vi "Joystick Read 1.vi"   [LabVIEW 2011]
uses:
  Robot Global Data.vi
types:
  T1 = typedef "WPI_JoystickDevRef.ctl" = cluster{"Device":T2}
  T2 = typedef "WPI_JoystickDeviceEnum.ctl" = enum16{"USB 1", "USB 2", "USB 3", "USB 4", "Kinect 1", "Kinect 2"}
  T3 = typedef "WPI_JoystickButtonState.ctl" = cluster{"Button 1":bool, "Button 2":bool, "Button 3":bool, "Button 4":bool, "Button 5":bool, "Button 6":bool, "Button 7":bool, "Button 8":bool, "Button 9":bool, "Button 10":bool, "Button 11":bool, "Button 12":bool}
  T4 = cluster{"axis 1 (x)":dbl, "axis 2 (y)":dbl, "axis 3 (throttle)":dbl, "axis 4":dbl, "axis 5":dbl, "axis 6":dbl}
  T5 = cluster{"Axis 1":dbl, "Axis 2":dbl, "Axis 3":dbl, "Axis 4":dbl, "Axis 5":dbl, "Axis 6":dbl, "Button 1":bool, "Button 2":bool, "Button 3":bool, "Button 4":bool, "Button 5":bool, "Button 6":bool, "Button 7":bool, "Button 8":bool, "Button 9":bool, "Button 10":bool, "Button 11":bool, "Button 12":bool}
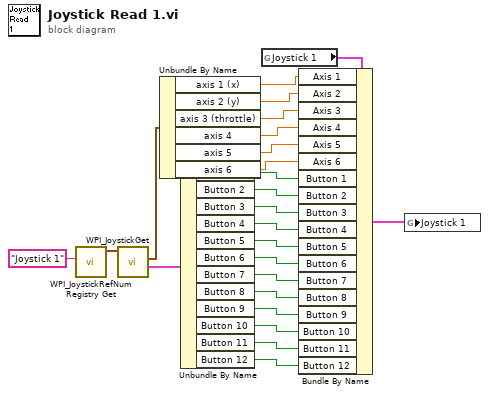
[diagram p0: block diagram]
diagram:
  n1 = call <vilib>:"WPI_JoystickRefNum Registry Get.vi"("refnum name"="Joystick 1") -> ("JoystickDevRef"=w23:T1)  [unwired: 1 in, 9 out]
  n2 = call <vilib>:"WPI_JoystickGet.vi"("JoystickDevRef"=w23) -> ("Buttons"=w21:T3, "Axes"=w22:T4)  [unwired: 1 in, 4 out]
  n3 = Unbundle By Name(w22) -> ("axis 1 (x)"=w19:dbl, "axis 2 (y)"=w18:dbl, "axis 3 (throttle)"=w17:dbl, "axis 4"=w16:dbl, "axis 5"=w15:dbl, "axis 6"=w14:dbl)
  n4 = Unbundle By Name(w21) -> ("Button 1"=w13:bool, "Button 2"=w12:bool, "Button 3"=w11:bool, "Button 4"=w10:bool, "Button 5"=w9:bool, "Button 6"=w8:bool, "Button 7"=w7:bool, "Button 8"=w6:bool, "Button 9"=w5:bool, "Button 10"=w4:bool, "Button 11"=w3:bool, "Button 12"=w2:bool)
  n5 = global read "Robot Global Data.vi" "Joystick 1"() -> (w1:T5)
  n6 = Bundle By Name(cluster=w1, "Axis 1"=w19, "Axis 2"=w18, "Axis 3"=w17, "Axis 4"=w16, "Axis 5"=w15, "Axis 6"=w14, "Button 1"=w13, "Button 2"=w12, "Button 3"=w11, "Button 4"=w10, "Button 5"=w9, "Button 6"=w8, "Button 7"=w7, "Button 8"=w6, "Button 9"=w5, "Button 10"=w4, "Button 11"=w3, "Button 12"=w2) -> (w20:T5)
  n7 = global write "Robot Global Data.vi" "Joystick 1"(w20) -> ()
